vi "限幅器（DBL）.vi"(3 "下限":dbl, 4 "X_in":dbl, 5 "上限":dbl) -> (1 "X_Out":dbl)   [LabVIEW 2012]
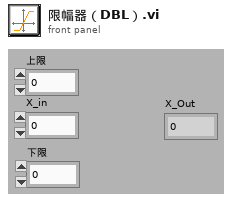
[diagram p1: front panel]
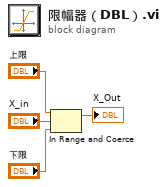
[diagram p0: block diagram]
diagram:
  n1 = In Range and Coerce ("判定范围并强制转换")(upper limit="上限", x="X_in", lower limit="下限") -> (coerced(x)=→"X_Out":dbl)  [unwired: 1 out]
